vi "Master Setup Read Write Convert Errors.vi"(8 "Reset":bool, 9 "Read (F) Write (T)":bool, 10 "Pattern Label":T1 items=["Channel Setup (0)", "PID Setup (1)", "Filter Setup (2)", "~Reserved Old CAN Msgs (3)", "~Reserved Old CAN1 (4)", "~Reserved Old CAN2 (5)", "Digital Inputs Setup (6)", "Digital Outputs Setup (7)", "Logging 1 Setup (8)", "Logging 2 Setup (9)", "Logging 3 Setup (10)", "Setpoint Setup (11)", "Test Series Setup (12)", "Graph Setup (13)", "System Configure (14)", "Header (15)", "Profile Manager (16)", "Post-Mortem Logging (17)", "High-Speed Data (18)", "Statistic Channel Setup (19)", "Ramp Channel Setup (20)", "ETAS INCA Channel Setup (21)", "ETC ECCS Transducer Setup (22)", "ETC ECCS Test Setup (23)", "AVL AK Smoke Meter Setup (24)", "Triggers Setup (25)", "Alarm Limits Setup (26)", "YKWT1 Measurement (27)", "YKWT1 Instrument (28)", "Auto File Settings (29)", "Playback File Setting (30)", "UUT Constants (31)", "UPS Setup (32)", "Differential Channel Setup (33)", "Integral Channel Setup (34)", "Signal Channel Setup (35)", "Calibration Setup (36)", "BNC Setup (37)", "ASAP3 Setup (38)", "Chassis Force Calculations (39)", "Chassis Teststand Losses (40)", "Chassis Vehicle Losses (41)", "Formula Channels (42)", "ASAP3 Map Coords Setup (43)", "Digital Controls Setup (44)", "Push Buttons Setup (45)", "Sliders Setup (46)", "~Reserved~ (47)", "Email Setup (48)", "Timer Setup (49)", "Unit Conversion Setup (50)", "Visible Channels (51)", "Main Display Setup (52)", "Message Display Setup (53)", "Input Display Setup (54)", "Unico Parameter Downloads (55)", "Flow Meter Setup (56)", "Channel Zero Offset (57)", "YKWT2 Measurement (58)", "YKWT2 Instrument (59)", "~Reserved Old CAN3 (60)", "CAS Setup (61)", "Accumulation Channel Setup (62)", "Valvetrain Dynamics Setup (63)", "CCP Setup (64)", "System Log Setup (65)", "Throttle Controller (66)", "RE Shifter (67)", "Main Display (68)", "~Reserved~ (69)", "FlexRay (70)", "YKWT3 Measurement (71)", "YKWT3 Instrument (72)", "CAN XNET API (73)"], 11 "Convert Error":errorcluster) -> (0 "error out (No Error)":errorcluster, 3 "Convert Error (out)":bool[](array[boolean]))   [LabVIEW 2017]
uses:
  Master Setup Pattern Enum.ctl
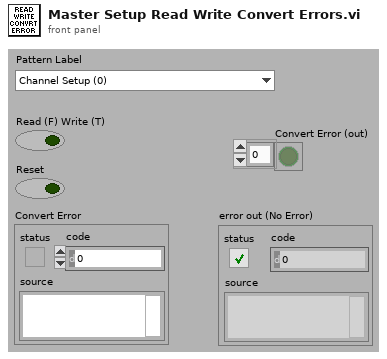
[diagram p1: front panel]
types:
  T1 = typedef "Master Setup Pattern Enum.ctl" = i32
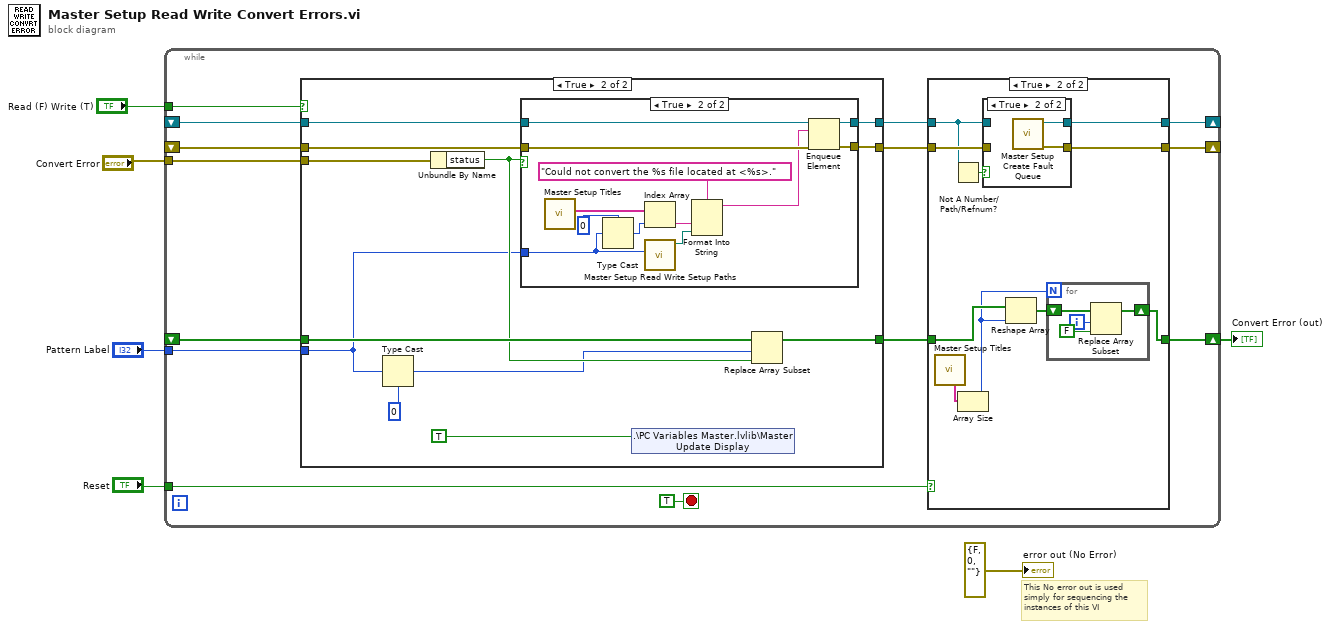
[diagram p0: block diagram]
diagram:
  # "This No error out is used\nsimply for sequencing the\ninstances of this VI"
  n1 = while {
    shift-right: [w19] -> w6
    shift-left: _ -> [w18]
    shift-right: [w16] -> _
    shift-left: _ -> [w14]
    shift-right: [w15] -> _
    shift-left: _ -> [w12]
    tunnel: "Convert Error" -> [w10]
    tunnel: "Read (F) Write (T)" -> [w9]
    tunnel: "Pattern Label" -> [w8]
    tunnel: "Reset" -> [w7]
    stop <- TRUE stop-if-true
    n2 = case shown="True" w9 {
      tunnel: [w23 w35] -> w17
      tunnel: w18 -> [w23 w34]
      tunnel: w8 -> [_ w24]
      tunnel: w14 -> [w22 w32]
      tunnel: [w22 w31] -> w13
      tunnel: w12 -> [w21 w30]
      tunnel: [w21 w29] -> w11
      tunnel: w10 -> [_ w27]
      frame False {
      }
      frame True {
        n3 = Type Cast(type=0, x=w24) -> (*(type *) &x=w25:i32)
        n4 = Unbundle By Name(w27) -> ("status"=w28:bool)
        n5 = case shown="True" w28 {
          tunnel: w32 -> [w37 w49]
          tunnel: [w37 w48] -> w31
          tunnel: w30 -> [w36 w47]
          tunnel: [w36 w46] -> w29
          tunnel: w24 -> [_ w38]
          frame False {
          }
          frame True {
            n6 = call "Master Setup Titles.vi"() -> ("Setup Description"=w45:string[])  [unwired: 6 in, 5 out]
            n7 = Type Cast(type=0, x=w38) -> (*(type *) &x=w39:i32)
            n8 = Index Array(array=w45, index=w39) -> (element=w43:string)
            n9 = call "Master Setup Read Write Setup Paths.vi"("Pattern Label"=w38) -> ("New Setup Path"=w42:path)  [unwired: 6 in, 4 out]
            n10 = Format Into String(format string="Could not convert the %s file located at <%s>." ("[Date/Time] [Fault Status] [Fault Type] ... [Channel Name] ... [Value] ... [Limit]"), w43, w42) -> (resulting string=w41:string)  [unwired: 2 in, 1 out]
            n11 = Enqueue Element(queue=w49, element=w41, error in (no error)=w47) -> (queue out=w48:refnum<queue>, error out=w46:errorcluster)  [unwired: 1 in, 1 out]
          }
        }
        n12 = shared-variable ".\\PC Variables Master.lvlib\\Master Update Display"(TRUE ("Master Update Display")) -> ()  [unwired: 1 in, 1 out]
        n13 = Replace Array Subset(array=w34, new element=w28, index=w25) -> (w35:bool[])
      }
    }
    n14 = case shown="True" w7 {
      tunnel: [w52 w54] -> w19
      tunnel: w17 -> [w52 w61]
      tunnel: [w51 w59] -> w16
      tunnel: w13 -> [w51 w56]
      tunnel: [w50 w58] -> w15
      tunnel: w11 -> [w50 w57]
      frame False {
      }
      frame True {
        n15 = call "Master Setup Titles.vi"() -> ("Sorted Setup Description"=w62:string[])  [unwired: 6 in, 5 out]
        n16 = Not A Number/Path/Refnum?(number/path/refnum=w56) -> (NaN/Path/Refnum?=w60:bool)
        n17 = Array Size(array=w62) -> (size(s)=w53:i32)
        n18 = case shown="True" w60 {
          tunnel: [w68 w70] -> w59
          tunnel: w56 -> [w68 _]
          tunnel: [w67 w69] -> w58
          tunnel: w57 -> [w67 _]
          frame False {
          }
          frame True {
            n19 = call "Master Setup Create Fault Queue.vi"() -> ("error out"=w69:errorcluster, "Master Fault Queue"=w70:refnum<queue>)  [unwired: 6 in]
          }
        }
        n20 = Reshape Array(w61, w53) -> (w55:bool[])
        n21 = for {
          N: w53 -> [_]
          shift-right: [w65] -> w54
          shift-left: w55 -> [w66]
          i -> [w63]
          n22 = Replace Array Subset(array=w66, new element=FALSE ("new element/subarray"), index=w63) -> (w65:bool[])
        }
      }
    }
  }
  "Convert Error (out)" <- w6
  "error out (No Error)" <- errorcluster {"status"=FALSE, "code"=0, "source"=""} ("error out (No Error)")
